vi "GyroSimulator.vi"() -> ()   [LabVIEW 2016]
uses:
  Common_FPGA_HealthAndStatus/DataTypes/HealthAndStatusFIFOCopySettings.ctl
  Common_FPGA_HealthAndStatus/DataTypes/HealthAndStatusSettings.ctl
  Common_FPGA_Timestamp/DataTypes/TimestampSettings.ctl
  Common_FPGA_Modbus/DataTypes/ModbusPortSettings.ctl
  FPGAMockGyro/DataTypes/MockGyroData.ctl
  <vilib>/rvi/Emulation/niFpgaGetClockAttributes.vi
  <vilib>/rvi/Emulation/niFpgaSctlEmulationGetInTimedLoop.vi
  <vilib>/rvi/Emulation/niFpgaEmulationReportErrorSimple.vi
  <vilib>/rvi/Memory/Memory_Emulation/nirvimemoryFastEmulation.vi
  <vilib>/rvi/Memory/Memory_Emulation/nirvimemoryEmulation.vi
  <vilib>/rvi/Emulation/niFpgaEmulationIsFPGAContextNoSignature.vi
  <vilib>/rvi/DataTransferAndStorage/Container/Common/niFpgaContainerGetUniqueNameForEmu.vi
  <vilib>/rvi/Emulation/niFpgaProcessEmulError.vi
  <vilib>/rvi/errors/nirviReportUnexpectedCaseInternalError (U32).vi
  <vilib>/rvi/DataTransferAndStorage/Container/Common/niFpgaContainerExecOnDevCompGetState.vi
  <vilib>/rvi/Memory/Memory_Emulation/niFpgaMemoryEmulationCacheClearOnFirstRun.vi
  <vilib>/rvi/Memory/Memory_Emulation/nirvimemoryEmulationManagerCache_MakeExclusive.vi
  <vilib>/rvi/Memory/Memory_Emulation/niFpgaMemoryEmulationValidateCache.vi
  <vilib>/rvi/Memory/Memory_Emulation/nirvimemoryEmulationManagerCache_InsertValue.vi
  <vilib>/Utility/error.llb/Clear Errors.vi
  <vilib>/rvi/Memory/Memory_Emulation/nirvimemoryEmulationManagerCache_ReleaseExclusive.vi
  <vilib>/rvi/Memory/Memory_Emulation/nirvimemoryEmulationManagerCache_GetValue.vi
  <vilib>/rvi/Memory/Memory_Emulation/nirvimemoryEmulationManagerCache_SetValue.vi
  <vilib>/rvi/Emulation/niFpgaSctlEmulationResourceMgr.vi
  <vilib>/rvi/Emulation/niFpgaCriticalErrorInLSC.vi
  <vilib>/rvi/eio/common/nirviEmuTemplateMethod_errors.vi
  <vilib>/rvi/errors/niFpgaSetErrorForExecOnDevCompSimple.vi
  <vilib>/rvi/eio/common/nirviEmuReportErrorAndStop.vi
  <vilib>/rvi/FIFO/Fifo_Resource/nirvififoEmulationSetSize.vi
  <vilib>/rvi/FIFO/Fifo_Resource/nirviFifoEmulationQueueMgr.vi
  <instcachedir>/0/nirviFifoEmulationQueueMgr_E5CAEC123FF24DC58D834DCA3CDAA9B5.lvgen/nirviFifoEmulationQueueMgr_E5CAEC123FF24DC58D834DCA3CDAA9B5_005.vi
  <vilib>/rvi/FIFO/Fifo_Resource/nirvififoEmulationCreateLock.vi
  <vilib>/rvi/FIFO/Fifo_Resource/nirvififoEmulationObtainLock.vi
  <vilib>/rvi/FIFO/Fifo_Resource/nirvififoEmulationReleaseLock.vi
  <vilib>/rvi/occurrence/nirviWaitOnOccurrenceBase.vi
  <vilib>/rvi/errors/nirviReportUnexpectedCaseInternalError.vi
  <vilib>/rvi/DataTransferAndStorage/Container/XNode/niFpgaContainer.xnode
  <vilib>/rvi/Memory/Memory_Emulation/niFpgaMemoryEmulationRefIn.vi
  <vilib>/eio/EIOMethodNode/EIOMethodNode.xnode
  <vilib>/rvi/FIFO/Fifo_Resource/nirvififoEmulationRead.vi
  FPGAMockGyro/FPGAMockGyro.lvlib
  Common_FPGA_HealthAndStatus/FPGAHealthAndStatus.lvlib
  Common_FPGA_Timestamp/FPGATimestamp.lvlib
  Common_FPGA_Modbus/FPGAModbus.lvlib
panel:
  out "GyroRxByteCount":u32
  out "GyroTxByteCount":u32
  out "GyroFlags":u32
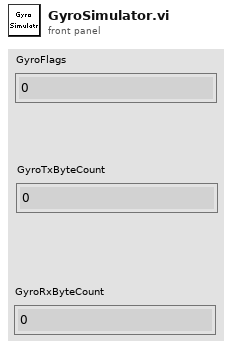
[diagram p1: front panel]
types:
  T1 = typedef "FPGAHealthAndStatus.lvlib/HealthAndStatusFIFOCopySettings.ctl" = cluster{"InternalHealthAndStatusFIFO":refnum<k21>, "SourceHealthAndStatusFIFO":refnum<k21>}
  T2 = typedef "FPGAMockGyro.lvlib/MockGyroData.ctl" = cluster{"BufferUpdateFIFO":refnum<k21>, "MockGyroCommandInput":refnum<k21>, "MockGyroDataOutput":refnum<k21>, "MockGyroDataRate":refnum<k21>, "MockGyroXValue":refnum<k21>, "MockGyroYValue":refnum<k21>, "MockGyroZValue":refnum<k21>, "MockGyroStatus":refnum<k21>, "MockGyroTemperature":refnum<k21>, "CRCDataFIFO":refnum<k21>, "CRCCalculateFIFO":refnum<k21>, "CRCFIFO":refnum<k21>, "MockGyroCommandReplyFIFO":refnum<k21>, "MockGyroReplyReadyFIFO":refnum<k21>, "MockGyroModeFIFO":refnum<k21>}
  T3 = typedef "FPGAModbus.lvlib/ModbusPortSettings.ctl" = cluster{"TxPort":refnum<k21>, "TxDataFIFO":refnum<k21>, "TxInternalDataFIFO":refnum<k21>, "TxHealthAndStatusFIFO":refnum<k21>, "RxPort":refnum<k21>, "RxDataFIFO":refnum<k21>, "RxHealthAndStatusFIFO":refnum<k21>, "WaitForRxFrameRegister":refnum<k21>, "BaseHealthAndStatusAddress":u32, "IRQAddress":u8, "TriggerIRQRegister":refnum<k21>, "SoftwareControlledTrigger":refnum<k21>, "TimestampRegister":refnum<k21>, "TxTimestampFIFO":refnum<k21>}
  T4 = typedef "FPGATimestamp.lvlib/TimestampSettings.ctl" = cluster{"TimeSource":refnum<k21>, "TimeRegister":refnum<k21>, "IterationsPerMicrosecond":i16, "UpdateFIFO":refnum<k21>, "HealthAndStatusFIFO":refnum<k21>, "HealthAndStatusAddress":i16, "IterationsPerHealthAndStatusUpdate":i16}
  T5 = typedef "FPGAHealthAndStatus.lvlib/HealthAndStatusSettings.ctl" = cluster{"InternalHealthAndStatusFIFO":refnum<k21>, "HealthAndStatusQueryFIFO":refnum<k21>, "HealthAndStatusResponseFIFO":refnum<k21>, "HealthAndStatusMemory":refnum<k21>, "MemorySize":i32}
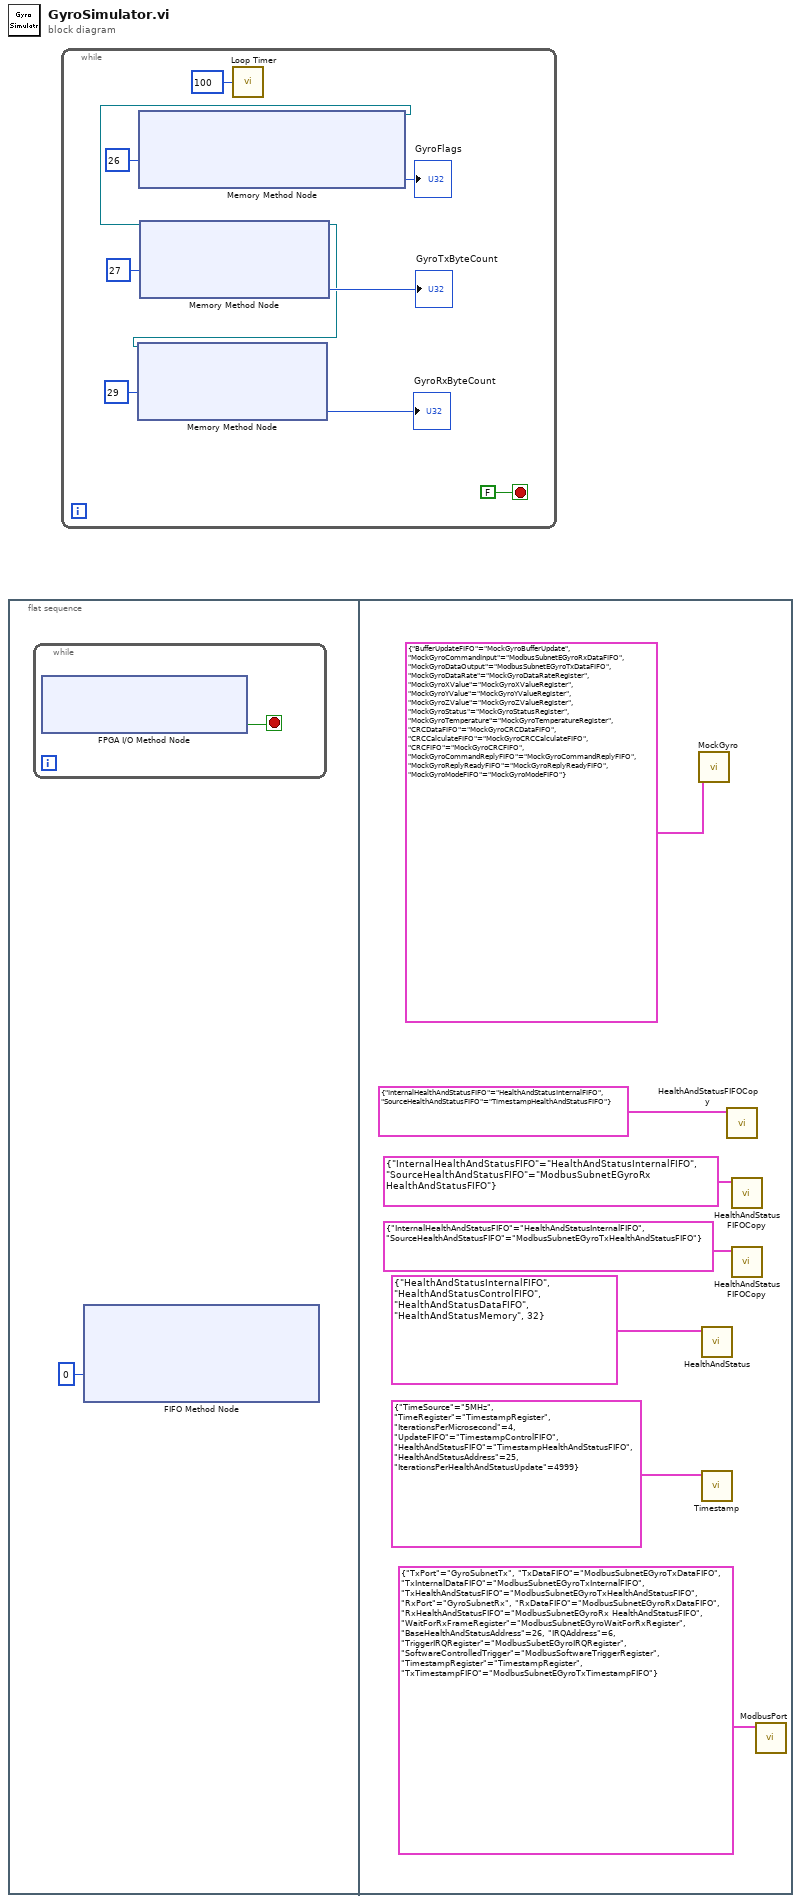
[diagram p0: block diagram]
diagram:
  n1 = flat-sequence {
    frame #0 {
      n2 = while {
        stop <- w2 stop-if-true
        n3 = xnode "FPGA I/O Method Node"() -> ("Ready"=w2:bool)  [unwired: 1 in, 1 out]
      }
      n4 = xnode ("FIFO Method Node")("Timeout"=0) -> ()  [unwired: 1 in, 3 out]
    }
    frame #1 {
      n5 = call "MockGyro.vi"("MockGyroData"=T2 {"BufferUpdateFIFO"="MockGyroBufferUpdate", "MockGyroCommandInput"="ModbusSubnetEGyroRxDataFIFO", "MockGyroDataOutput"="ModbusSubnetEGyroTxDataFIFO", "MockGyroDataRate"="MockGyroDataRateRegister", "MockGyroXValue"="MockGyroXValueRegister", "MockGyroYValue"="MockGyroYValueRegister", "MockGyroZValue"="MockGyroZValueRegister", "MockGyroStatus"="MockGyroStatusRegister", "MockGyroTemperature"="MockGyroTemperatureRegister", "CRCDataFIFO"="MockGyroCRCDataFIFO", "CRCCalculateFIFO"="MockGyroCRCCalculateFIFO", "CRCFIFO"="MockGyroCRCFIFO", "MockGyroCommandReplyFIFO"="MockGyroCommandReplyFIFO", "MockGyroReplyReadyFIFO"="MockGyroReplyReadyFIFO", "MockGyroModeFIFO"="MockGyroModeFIFO"}) -> ()  [unwired: 11 in]
      n6 = call "HealthAndStatus.vi"("HealthAndStatusSettings"=T5 {"InternalHealthAndStatusFIFO"="HealthAndStatusInternalFIFO", "HealthAndStatusQueryFIFO"="HealthAndStatusControlFIFO", "HealthAndStatusResponseFIFO"="HealthAndStatusDataFIFO", "HealthAndStatusMemory"="HealthAndStatusMemory", "MemorySize"=32}) -> ()  [unwired: 11 in]
      n7 = call "Timestamp.vi"("TimestampSettings"=T4 {"TimeSource"="5MHz", "TimeRegister"="TimestampRegister", "IterationsPerMicrosecond"=4, "UpdateFIFO"="TimestampControlFIFO", "HealthAndStatusFIFO"="TimestampHealthAndStatusFIFO", "HealthAndStatusAddress"=25, "IterationsPerHealthAndStatusUpdate"=4999}) -> ()  [unwired: 11 in]
      n8 = call "HealthAndStatusFIFOCopy.vi"("HealthAndStatusSettingsFIFOCopySettings"=T1 {"InternalHealthAndStatusFIFO"="HealthAndStatusInternalFIFO", "SourceHealthAndStatusFIFO"="TimestampHealthAndStatusFIFO"}) -> ()  [unwired: 11 in]
      n9 = call "HealthAndStatusFIFOCopy.vi"("HealthAndStatusSettingsFIFOCopySettings"=T1 {"InternalHealthAndStatusFIFO"="HealthAndStatusInternalFIFO", "SourceHealthAndStatusFIFO"="ModbusSubnetEGyroRx HealthAndStatusFIFO"}) -> ()  [unwired: 11 in]
      n10 = call "HealthAndStatusFIFOCopy.vi"("HealthAndStatusSettingsFIFOCopySettings"=T1 {"InternalHealthAndStatusFIFO"="HealthAndStatusInternalFIFO", "SourceHealthAndStatusFIFO"="ModbusSubnetEGyroTxHealthAndStatusFIFO"}) -> ()  [unwired: 11 in]
      n11 = call "ModbusPort.vi"("ModbusPortSettings"=T3 {"TxPort"="GyroSubnetTx", "TxDataFIFO"="ModbusSubnetEGyroTxDataFIFO", "TxInternalDataFIFO"="ModbusSubnetEGyroTxInternalFIFO", "TxHealthAndStatusFIFO"="ModbusSubnetEGyroTxHealthAndStatusFIFO", "RxPort"="GyroSubnetRx", "RxDataFIFO"="ModbusSubnetEGyroRxDataFIFO", "RxHealthAndStatusFIFO"="ModbusSubnetEGyroRx HealthAndStatusFIFO", "WaitForRxFrameRegister"="ModbusSubnetEGyroWaitForRxRegister", "BaseHealthAndStatusAddress"=26, "IRQAddress"=6, "TriggerIRQRegister"="ModbusSubetEGyroIRQRegister", "SoftwareControlledTrigger"="ModbusSoftwareTriggerRegister", "TimestampRegister"="TimestampRegister", "TxTimestampFIFO"="ModbusSubnetEGyroTxTimestampFIFO"}) -> ()  [unwired: 10 in]
    }
  }
  n12 = while {
    stop <- FALSE stop-if-true
    n13 = xnode ("Memory Method Node")("Address"=u32 26) -> ("Data"=→"GyroFlags":u32, "Memory Out"=w11:refnum<k21>)  [unwired: 1 in]
    n14 = xnode ("Memory Method Node")("Address"=u32 27, "Memory In"=w11) -> ("Data"=→"GyroTxByteCount":u32, "Memory Out"=w10:refnum<k21>)
    n15 = xnode ("Memory Method Node")("Address"=u32 29, "Memory In"=w10) -> ("Data"=→"GyroRxByteCount":u32)  [unwired: 1 out]
    n16 = call "Loop Timer"("Count(mSec)"=u32 100) -> ()  [unwired: 1 out]
  }
